vi "Main.vi"() -> ()   [LabVIEW 2018]
uses:
  <vilib>/smtpClient/Set Message Text.vi
  <vilib>/smtpClient/LabVIEWSMTPClient.lvlib
panel:
  in  "Face Presence Code path":path
  in  "Stop (F)":bool
  out "Image Out 2":T1(plugin-control)
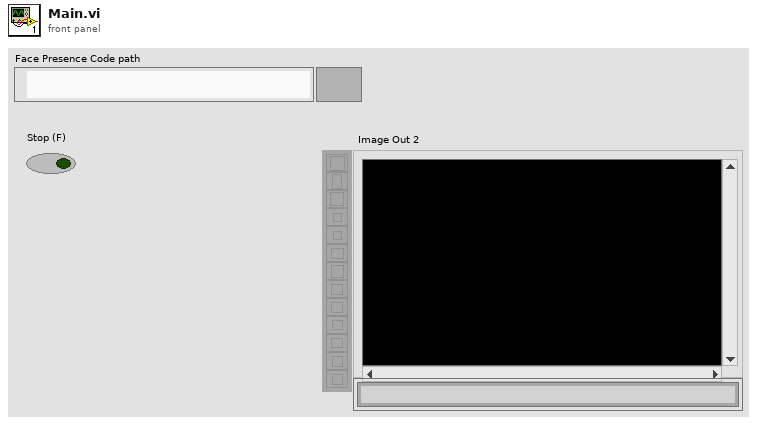
[diagram p1: front panel]
types:
  T1 = typedef "IMAQ Image.ctl" = refnum<image>
  T2 = typedef "LabVIEWSMTPClient.lvlib/SmtpClientHandle.ctl" = refnum<k1>
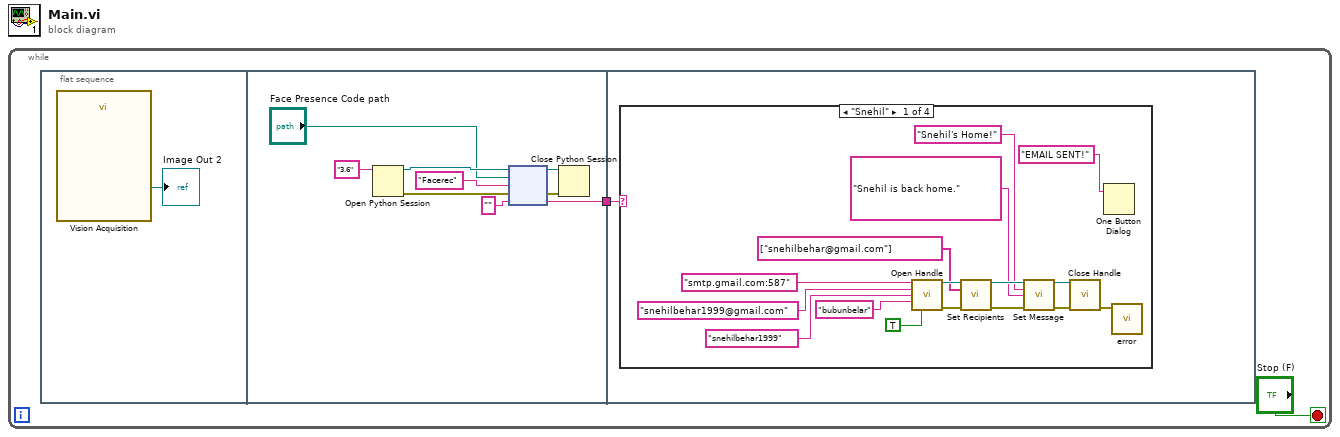
[diagram p0: block diagram]
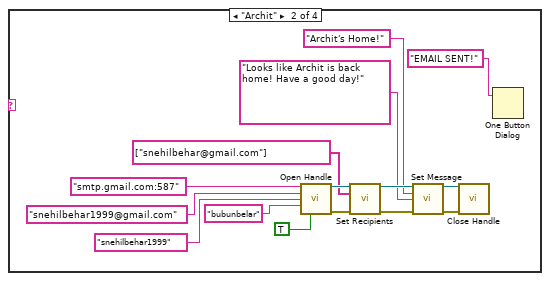
[diagram p2: hidden frame]
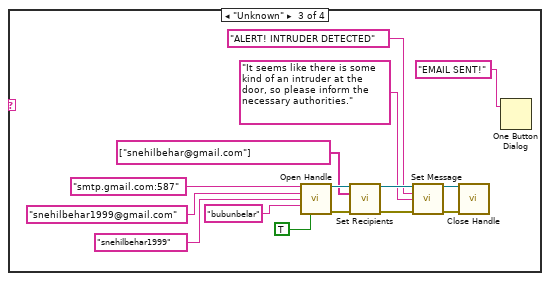
[diagram p3: hidden frame]
diagram:
  n1 = while {
    stop <- "Stop (F)" stop-if-true
    n2 = flat-sequence {
      tunnel: [w5] -> w1
      tunnel: w1 -> [w13]
      frame #0 {
        n3 = call "Vision Acquisition"() -> ("Image Out"=→"Image Out 2":T1)  [unwired: 26 in, 1 out]
      }
      frame #1 {
        n4 = Open Python Session(python version="3.6" ("Python version")) -> (session out=w11:refnum<k35>, error out=w8:errorcluster)  [unwired: 2 in]
        n5 = node(w11, "Face Presence Code path", "Facerec" ("function name"), w8, "") -> (w10:refnum<k35>, w7:errorcluster, w5:string)  [unwired: 2 out]
        n6 = Close Python Session(session in=w10, error in=w7) -> ()  [unwired: 1 out]
      }
      frame #2 {
        n7 = case shown="\"Snehil\"" w13 {
          frame "Snehil" {
            n8 = call <vilib>:"Open Handle.vi"("server address"="smtp.gmail.com:587", "from"="snehilbehar1999@gmail.com", "username"="snehilbehar1999", "password"="bubunbelar", "use TLS (false)"=TRUE) -> ("handle out"=w25:T2, "error out"=w22:errorcluster)  [unwired: 9 in]
            n9 = call <vilib>:"Set Recipients.vi"("handle in"=w25, "to"=string[] ["snehilbehar@gmail.com"], "error in (no error)"=w22) -> ("handle out"=w24:T2, "error out"=w23:errorcluster)  [unwired: 11 in]
            n10 = call-poly <vilib>:"Set Message.vi"("handle in"=w24, "subject"="Snehil's Home!", "plain text message"="Snehil is back home.", "error in (no error)"=w23) -> ("handle out"=w18:T2, "error out"=w17:errorcluster)  [unwired: 10 in]
            n11 = call <vilib>:"Close Handle.vi"("handle in"=w18, "error in (no error)"=w17) -> ("error out"=w15:errorcluster)  [unwired: 12 in, 1 out]
            n12 = One Button Dialog(message="EMAIL SENT!") -> ()  [unwired: 1 in, 1 out]
            n13 = call "error.vi"("error in (no error)"=w15) -> ()  [unwired: 11 in]
          }
          frame "Archit" {
            n14 = call <vilib>:"Open Handle.vi"("server address"="smtp.gmail.com:587", "from"="snehilbehar1999@gmail.com", "username"="snehilbehar1999", "password"="bubunbelar", "use TLS (false)"=TRUE) -> ("handle out"=w40:T2, "error out"=w37:errorcluster)  [unwired: 9 in]
            n15 = call <vilib>:"Set Recipients.vi"("handle in"=w40, "to"=string[] ["snehilbehar@gmail.com"], "error in (no error)"=w37) -> ("handle out"=w39:T2, "error out"=w38:errorcluster)  [unwired: 11 in]
            n16 = call-poly <vilib>:"Set Message.vi"("handle in"=w39, "subject"="Archit's Home!", "plain text message"="Looks like Archit is back home! Have a good day!", "error in (no error)"=w38) -> ("handle out"=w33:T2, "error out"=w32:errorcluster)  [unwired: 10 in]
            n17 = call <vilib>:"Close Handle.vi"("handle in"=w33, "error in (no error)"=w32) -> ()  [unwired: 12 in, 2 out]
            n18 = One Button Dialog(message="EMAIL SENT!") -> ()  [unwired: 1 in, 1 out]
          }
          frame "Unknown" {
            n19 = call <vilib>:"Open Handle.vi"("server address"="smtp.gmail.com:587", "from"="snehilbehar1999@gmail.com", "username"="snehilbehar1999", "password"="bubunbelar", "use TLS (false)"=TRUE) -> ("handle out"=w55:T2, "error out"=w52:errorcluster)  [unwired: 9 in]
            n20 = call <vilib>:"Set Recipients.vi"("handle in"=w55, "to"=string[] ["snehilbehar@gmail.com"], "error in (no error)"=w52) -> ("handle out"=w54:T2, "error out"=w53:errorcluster)  [unwired: 11 in]
            n21 = call-poly <vilib>:"Set Message.vi"("handle in"=w54, "subject"="ALERT! INTRUDER DETECTED", "plain text message"="It seems like there is some kind of an intruder at the door, so please inform the necessary authorities.", "error in (no error)"=w53) -> ("handle out"=w48:T2, "error out"=w47:errorcluster)  [unwired: 10 in]
            n22 = call <vilib>:"Close Handle.vi"("handle in"=w48, "error in (no error)"=w47) -> ()  [unwired: 12 in, 2 out]
            n23 = One Button Dialog(message="EMAIL SENT!") -> ()  [unwired: 1 in, 1 out]
          }
          frame Default {
          }
        }
      }
    }
  }
